vi "EventLog.Buffer.Reload.vi"(8 "error in":errorcluster, 11 "Path":path) -> (0 "error out":errorcluster)   [LabVIEW 2016]
uses:
  EventLog.Buffer.Action.ctl
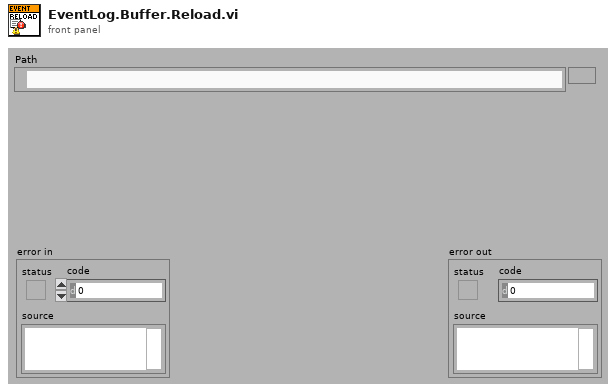
[diagram p1: front panel]
types:
  T1 = typedef "EventLog.Buffer.Action.ctl" = enum16{"init", "re-init", "clear", "set translator", "translate", "add", "get"}
  T2 = typedef "EventLog.EventGui.ctl" = cluster{"ts":dbl, "lev":T3, "src":T4, "msg":T5, "arg":variant[], "msg_str":string}
  T3 = typedef "EventLog.EventLevel.ctl" = enum8{"Debug", "Info", "Warning", "Error"}
  T4 = typedef "EventLog.EventSource.ctl" = enum16{"All", "Gui", "Cache", "PLC1", "PLC2", "PLC3", "DB", "DB01", "DB02", "DB03", "DB04", "DB05", "DB06", "DB07", "DB08", "DB09", "DB10", "DB11", "DB12", "DB13", "DB14", "DB15", "DB16"}
  T5 = typedef "Translator.Message.ctl" = enum16{"-", "Event confirmed", "Log out", "Log in", "Shutdown", "Cancel", "Start", "Continue", "Stop", "On", "Off", "OK", "NOK", "NOK %s", "This", "Prev", "Home", "Work", "In progress...", "Missing", "Empty", "Hardware failure", "Initial", "Error %d >> %s", "Error %d >> %s >> %s", "Starting %s", "Quitting %s", "Configured", "Initializing", "Quitting", "Loading", "Running %s", "Stopped", "Summary", "Do you want to continue?", "Do you want to exit?", "Log out?", "System", "All", "IDLE", "Translating...%s", "Not found", "Alarm %s", "Run", "Skip", "Abort", "Repeat", "Please wait...", "Database disconnected", "Login to database successful", "Login to database failed: %d; %s", "Get process step data for %s", "Changeover off", "Changeover into %s", "Product %s | %s found in cache with status %d at previous station", "Product %s | %s found in database with status %d at previous station", "Product %s | %s not found in cache at previous station", "Product %s | %s not found in database at previous station", "Product %s | %s found in cache with status %d at this station (%d repetion)", "Product %s | %s found in database with status %d at this station (%d repetition)", "Product %s | %s not found in cache at this station", "Product %s | %s not found in database at this station", "Product %s | %s found in cache for component %s | %s", "Product %s | %s found in database for component %s | %s", "Product not found in cache for component %s | %s", "Product not found in database for component %s | %s", "Product %s | %s connected with component %s | %s (cache)", "Product %s | %s connected with component %s | %s (database)", "New data for %s | %s (cache)", "New data for %s | %s (database)", "File %s moved (cache)", "File %s deleted (cache)", "Msg %d >> %s", "PLC LifeBit Failure", "Reconnecting DB", "Reconnecting PLC", "Free disk space is below 1GB - contact technician", "Unable to check product status", "Product %s SN %s checked in DB", "Unable To check status from station %s"}
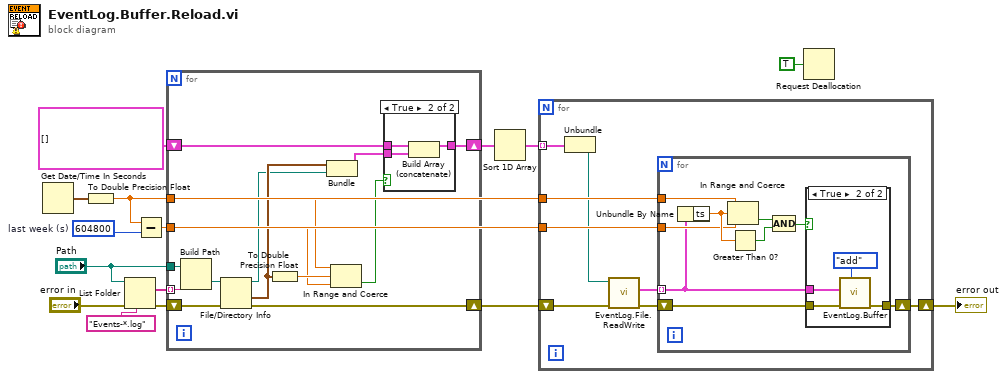
[diagram p0: block diagram]
diagram:
  w12 = 604800  # last week (s)
  n1 = Get Date/Time In Seconds() -> (seconds since 1Jan1904=w1:timestamp)
  n2 = To Double Precision Float(number=w1) -> (double precision float=w8:dbl)
  n3 = List Folder(path="Path", pattern="Events-*.log", error in="error in") -> (filenames=w4:string[], error out=w3:errorcluster)  [unwired: 1 in, 2 out]
  n4 = Subtract(x=w8, y=w12) -> (x-y=w7:dbl)
  n5 = for {
    tunnel: "Path" -> [w18]
    tunnel: w8 -> [w20]
    tunnel: w7 -> [w19]
    shift-right: [w28] -> w13
    shift-left: cluster{"last mod":timestamp, "path out":path}[] [] ("Chart file names in use") -> [w29]
    tunnel: w4 -> [w16] mode=indexing
    shift-right: [w21] -> w11
    shift-left: w3 -> [w27]
    n6 = Build Path(base path=w18, name or relative path=w16) -> (appended path=w17:path)
    n7 = File/Directory Info(path=w17, error in=w27) -> (path out=w23:path, last mod=w24:timestamp, error out=w21:errorcluster)  [unwired: 4 out]
    n8 = To Double Precision Float(number=w24) -> (double precision float=w26:dbl)
    n9 = Bundle("last mod"=w24, "path out"=w23) -> (w22:cluster{"last mod":timestamp, "path out":path})  [unwired: 1 in]
    n10 = In Range and Coerce(upper limit=w20, x=w26, lower limit=w19) -> (In Range?=w25:bool)  [unwired: 1 out]
    n11 = case shown="True" w25 {
      tunnel: w29 -> [w30 w33]
      tunnel: [w30 w32] -> w28
      tunnel: w22 -> [_ w31]
      frame False {
      }
      frame True {
        n12 = Build Array (concatenate)(w33, w31) -> (w32:cluster{"last mod":timestamp, "path out":path}[])
      }
    }
  }
  n13 = Sort 1D Array(array=w13) -> (sorted array=w9:cluster{"last mod":timestamp, "path out":path}[])
  n14 = for {
    shift-right: [w40] -> w10
    shift-left: w11 -> [w37]
    tunnel: w9 -> [w41] mode=indexing
    tunnel: w8 -> [w39]
    tunnel: w7 -> [w38]
    n15 = Unbundle(w41) -> ("path out"=w34:path)  [unwired: 1 out]
    n16 = call "EventLog.File.ReadWrite.vi"("error in"=w37, "file"=w34) -> ("error out"=w36:errorcluster, "Events out"=w35:T2[])  [unwired: 5 in, 3 out]
    n17 = for {
      tunnel: w35 -> [w42] mode=indexing
      tunnel: w39 -> [w47]
      tunnel: w38 -> [w46]
      shift-right: [w43] -> w40
      shift-left: w36 -> [w44]
      n18 = Unbundle By Name(w42) -> ("ts"=w48:dbl)
      n19 = In Range and Coerce(upper limit=w47, x=w48, lower limit=w46) -> (In Range?=w50:bool)  [unwired: 1 out]
      n20 = Greater Than 0?(x=w48) -> (x > 0?=w49:bool)
      n21 = Compound Arithmetic op=AND(w50, w49) -> (w45:bool)
      n22 = case shown="True" w45 {
        tunnel: w44 -> [w51 w54]
        tunnel: [w51 w53] -> w43
        tunnel: w42 -> [_ w52]
        frame False {
        }
        frame True {
          n23 = call "EventLog.Buffer.vi"("action (get)"=EventLog.Buffer.Action."add" ("action (read)"), "error in"=w54, "Event in"=w52) -> ("error out"=w53:errorcluster)  [unwired: 5 in, 3 out]
        }
      }
    }
  }
  "error out" <- w10
  n24 = Request Deallocation(TRUE ("flag")) -> ()
